vi "Scada.vi"() -> ()   [LabVIEW 2015]
uses:
  Controls Type/square.ctl
panel:
  in  "显示禁用":bool=TRUE
  in  "02-01":bool
  in  "02-02":bool
  in  "01-31":bool
  in  "02-11":bool
  in  "02-03":bool
  in  "02-09":bool
  in  "02-08":bool
  in  "02-07":T1
  in  "02-06":bool
  in  "02-05":bool
  in  "02-04":bool
  in  "02-15":bool
  in  "02-14":T1
  in  "02-13":bool
  in  "02-12":bool
  in  "02-10":T1
  in  "01-30":bool
  in  "01-29":T1
  in  "01-28":bool
  in  "01-27":bool
  in  "01-26":T1
  in  "01-25":bool
  in  "01-24":bool
  in  "01-23":bool
  in  "01-22":T1
  in  "01-21":bool
  in  "01-20":T1
  in  "01-19":bool
  in  "01-18":bool
  in  "01-17":T1
  in  "01-15":bool
  in  "01-14":T1
  in  "01-13":bool
  in  "01-12":bool
  in  "01-11":bool
  in  "01-10":T1
  in  "01-09":bool
  in  "01-08":bool
  in  "01-07":bool
  in  "01-06":bool
  in  "01-05":bool
  in  "01-04":bool
  in  "01-03":bool
  in  "01-02":bool
  in  "01-01":bool
  out "时间":string="14 : 47 : 23" caption="天"
  out "星期":string caption="星\n期"
  out "日":string caption="天"
  out "年":string caption="天"
  out "月":string caption="天"
  out "安全运行":string caption="天"
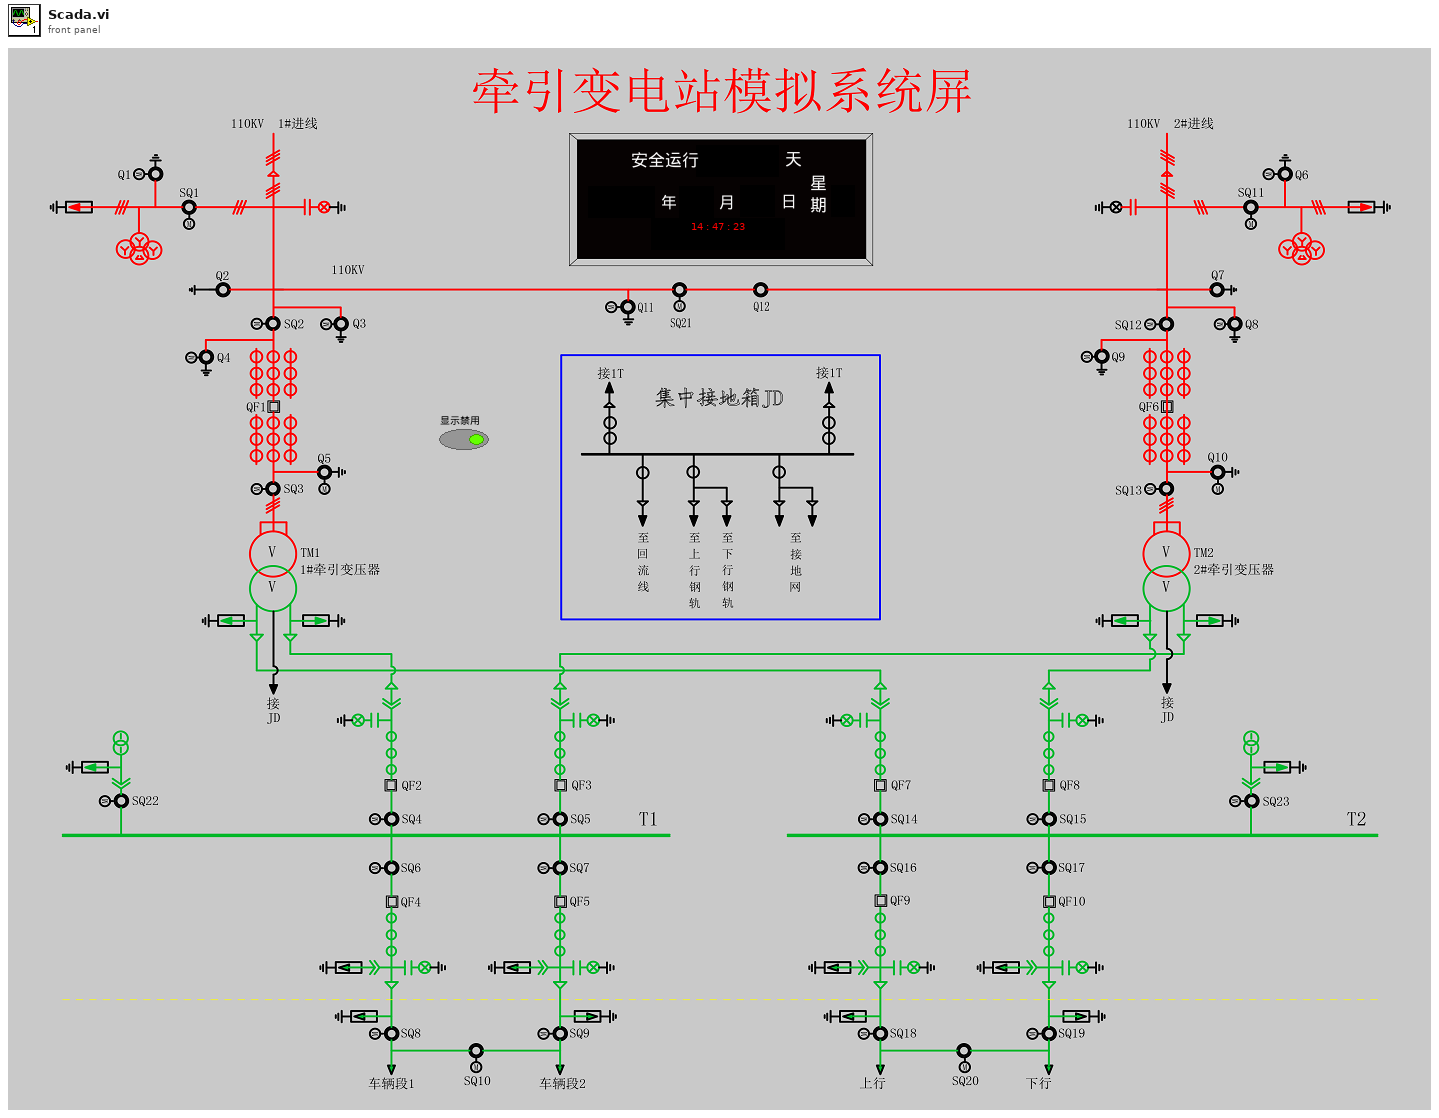
[diagram p1: front panel]
types:
  T1 = typedef "square.ctl" = bool
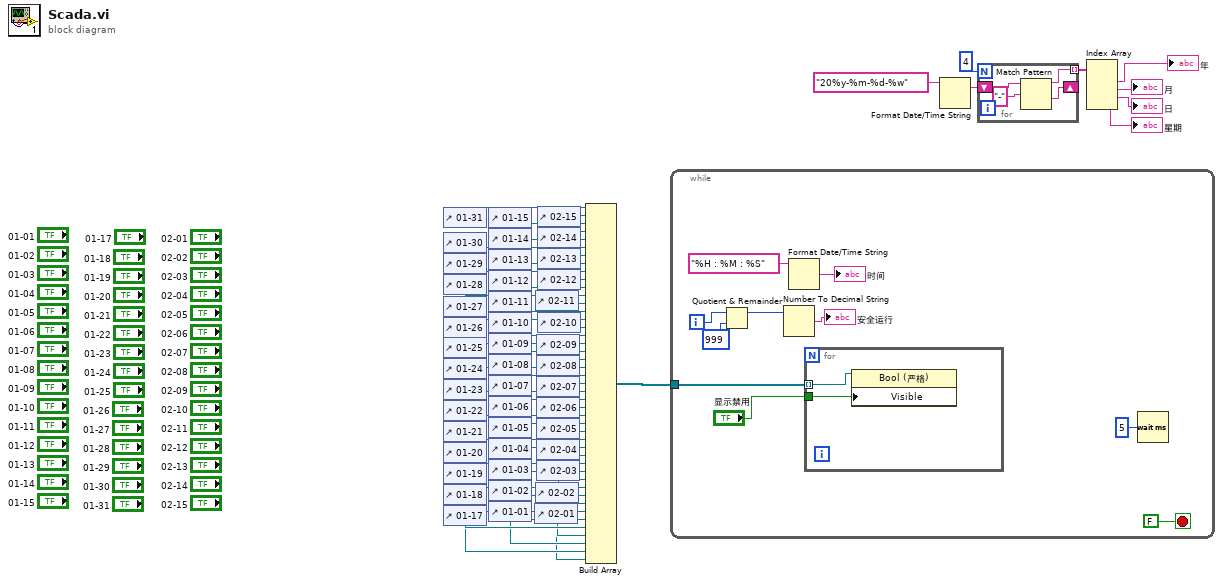
[diagram p0: block diagram]
diagram:
  n1 = control-ref of="01-31"() -> (w54:refnum<vi>)
  n2 = control-ref of="01-30"() -> (w49:refnum<vi>)
  n3 = control-ref of="01-29"() -> (w46:refnum<vi>)
  n4 = control-ref of="01-28"() -> (w43:refnum<vi>)
  n5 = control-ref of="01-27"() -> (w40:refnum<vi>)
  n6 = control-ref of="01-26"() -> (w37:refnum<vi>)
  n7 = control-ref of="01-25"() -> (w34:refnum<vi>)
  n8 = control-ref of="01-24"() -> (w31:refnum<vi>)
  n9 = control-ref of="01-23"() -> (w28:refnum<vi>)
  n10 = control-ref of="01-22"() -> (w25:refnum<vi>)
  n11 = control-ref of="01-21"() -> (w22:refnum<vi>)
  n12 = control-ref of="01-20"() -> (w19:refnum<vi>)
  n13 = control-ref of="01-19"() -> (w16:refnum<vi>)
  n14 = control-ref of="01-18"() -> (w14:refnum<vi>)
  n15 = control-ref of="01-17"() -> (w11:refnum<vi>)
  n16 = control-ref of="01-15"() -> (w52:refnum<vi>)
  n17 = control-ref of="01-14"() -> (w50:refnum<vi>)
  n18 = control-ref of="01-13"() -> (w47:refnum<vi>)
  n19 = control-ref of="01-12"() -> (w44:refnum<vi>)
  n20 = control-ref of="01-11"() -> (w41:refnum<vi>)
  n21 = control-ref of="01-10"() -> (w38:refnum<vi>)
  n22 = control-ref of="01-09"() -> (w36:refnum<vi>)
  n23 = control-ref of="01-08"() -> (w33:refnum<vi>)
  n24 = control-ref of="01-07"() -> (w30:refnum<vi>)
  n25 = control-ref of="01-06"() -> (w27:refnum<vi>)
  n26 = control-ref of="01-05"() -> (w24:refnum<vi>)
  n27 = control-ref of="01-04"() -> (w21:refnum<vi>)
  n28 = control-ref of="01-03"() -> (w18:refnum<vi>)
  n29 = control-ref of="01-02"() -> (w15:refnum<vi>)
  n30 = control-ref of="01-01"() -> (w12:refnum<vi>)
  n31 = control-ref of="02-01"() -> (w10:refnum<vi>)
  n32 = control-ref of="02-11"() -> (w42:refnum<vi>)
  n33 = control-ref of="02-02"() -> (w13:refnum<vi>)
  n34 = control-ref of="02-09"() -> (w35:refnum<vi>)
  n35 = control-ref of="02-08"() -> (w32:refnum<vi>)
  n36 = control-ref of="02-07"() -> (w29:refnum<vi>)
  n37 = control-ref of="02-06"() -> (w26:refnum<vi>)
  n38 = control-ref of="02-05"() -> (w23:refnum<vi>)
  n39 = control-ref of="02-04"() -> (w20:refnum<vi>)
  n40 = control-ref of="02-03"() -> (w17:refnum<vi>)
  n41 = control-ref of="02-15"() -> (w53:refnum<vi>)
  n42 = control-ref of="02-14"() -> (w51:refnum<vi>)
  n43 = control-ref of="02-13"() -> (w48:refnum<vi>)
  n44 = control-ref of="02-12"() -> (w45:refnum<vi>)
  n45 = control-ref of="02-10"() -> (w39:refnum<vi>)
  n46 = Build Array(w54, w53, w52, w51, w50, w49, w48, w47, w46, w45, w44, w43, w42, w41, w40, w39, w38, w37, w36, w35, w34, w33, w32, w31, w30, w29, w28, w27, w26, w25, w24, w23, w22, w21, w20, w19, w18, w17, w16, w15, w14, w13, w12, w11, w10) -> (w9:refnum<vi>[])
  n47 = while {
    tunnel: w9 -> [w62]
    i -> [w57]
    stop <- FALSE stop-if-true
    n48 = Quotient & Remainder(x=w57, y=999) -> (x-y*floor(x/y)=w55:i32)  [unwired: 1 out]
    n49 = Number To Decimal String(number=w55) -> (decimal integer string=→"安全运行":string)  [unwired: 1 in]
    n50 = Format Date/Time String(time format string (%c)="%H : %M : %S" ("时间格式字符串(%c)")) -> (date/time string=→"时间":string)  [unwired: 2 in]
    n51 = for {
      tunnel: w62 -> [w66] mode=indexing
      tunnel: "显示禁用" -> [w65]
      n52 = property class="Bool (严格)"(reference=w66, "Visible"=w65) -> ()  [unwired: 1 in, 2 out]
    }
    n53 = Wait (ms)(milliseconds to wait=u32 5 ("等待时间（毫秒）")) -> ()  [unwired: 1 out]
  }
  n54 = Format Date/Time String(time format string (%c)="20%y-%m-%d-%w" ("时间格式字符串(%c)")) -> (date/time string=w4:string)  [unwired: 2 in]
  n55 = for {
    N: 4 -> [_]
    shift-right: [w68] -> _
    shift-left: w4 -> [w69]
    tunnel: [w67] -> w6 mode=indexing
    n56 = Match Pattern(string=w69, regular expression="-" ("正则表达式")) -> (before substring=w67:string, after substring=w68:string)  [unwired: 1 in, 2 out]
  }
  n57 = Index Array(array=w6) -> (element #1=→"年":string, element #2=→"月":string, element #3=→"日":string, element #4=→"星期":string)  [unwired: 4 in]
